vi "WILT Watering Times.vi"(5 "Watering Times Input":T3, 7 "Execution Type":enum16{"Write", "Read"}(ring), 8 "Error In":errorcluster, 11 "File Locations":T1[](array[typedef])) -> (0 "Error Out":errorcluster, 3 "Watering Times Output":T3)   [LabVIEW 2016]
uses:
  Type Definitions/WILT Injection Times.ctl
  Type Definitions/WILT Water Injection Control.ctl
  Utility/Save File/File Setup (Public)/Type Definition/Save File DOE File Path Control.ctl
  Utility/Save File/File Setup (Public)/Type Definition/Save File DOE Data Save Filepaths.ctl
  <vilib>/Utility/file.llb/Write To Spreadsheet File (string).vi
  <vilib>/Utility/file.llb/Read From Spreadsheet File (string).vi
  Utility/Save File/File Setup.lvlib
panel:
  out "all rows":string[][](array[string])
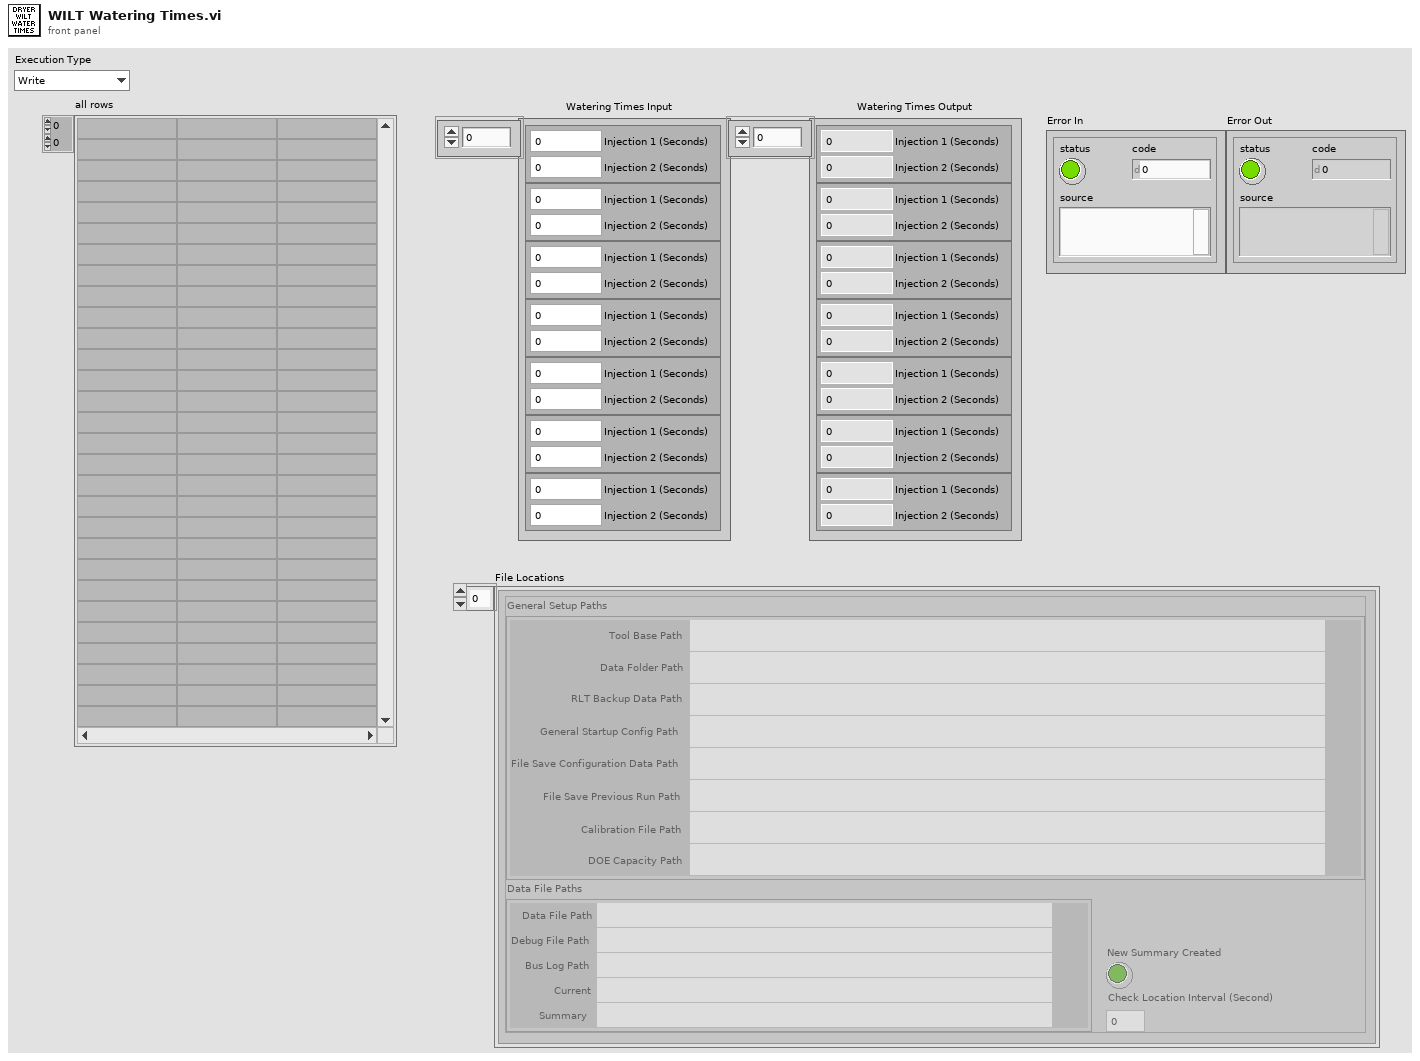
[diagram p1: front panel]
types:
  T1 = typedef "File Setup.lvlib/Save File DOE File Path Control.ctl" = cluster{"General Setup Paths":cluster{"Calibration File Path":path, "DOE Capacity Path":path, "Data Folder Path":path, "RLT Backup Data Path":path, "Tool Base Path":path, "General Startup Config Path":path, "File Save Previous Run Path":path, "File Save Configuration Data Path":path}, "Data File Paths":T2, "New Summary Created":bool, "Check Location Interval (Second)":i32}
  T2 = typedef "File Setup.lvlib/Save File DOE Data Save Filepaths.ctl" = cluster{"Data File Path":path, "Debug File Path":path, "Bus Log Path":path, "Current":path, "Summary":path}
  T3 = typedef "WILT Injection Times.ctl" = T4[]
  T4 = typedef "WILT Water Injection Control.ctl" = cluster{"Injection 1 (Seconds)":dbl, "Injection 2 (Seconds)":dbl}
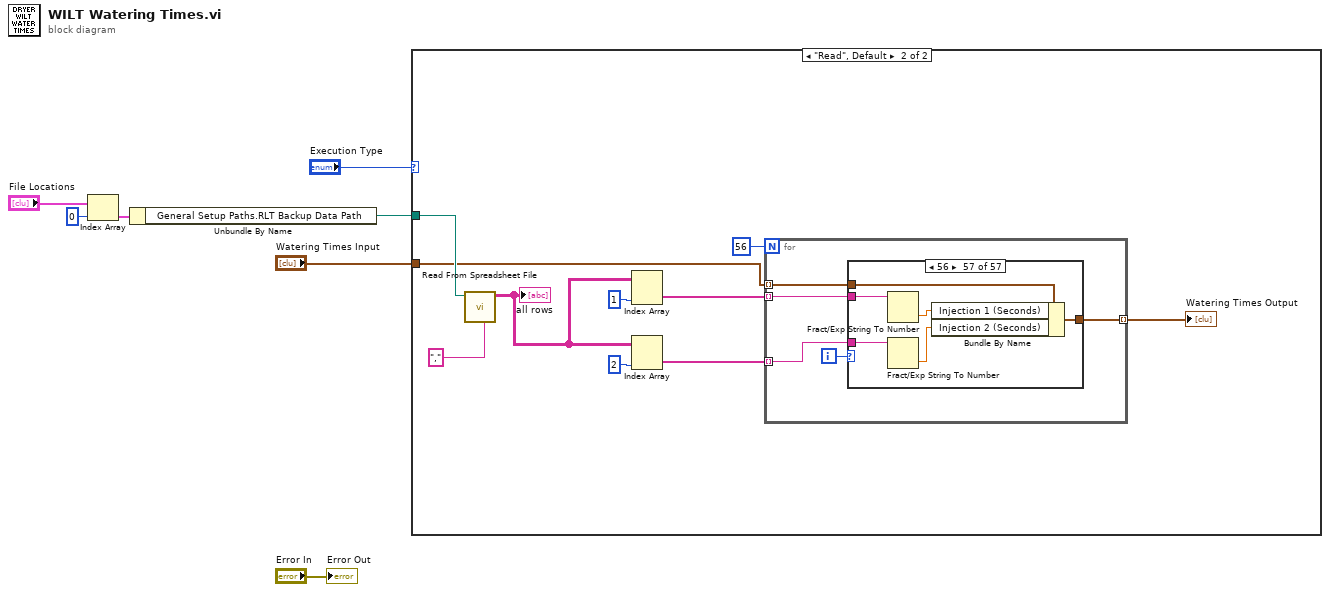
[diagram p0: block diagram]
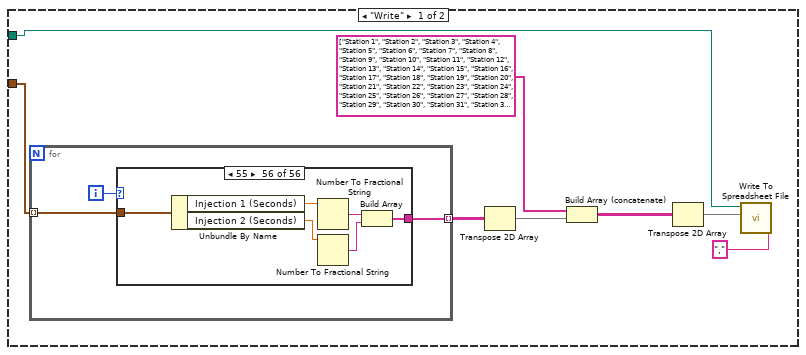
[diagram p2: hidden frame]
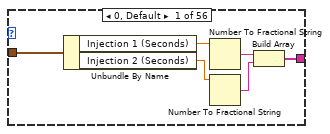
[diagram p3: hidden frame]
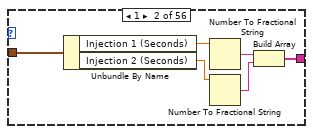
[diagram p4: hidden frame]
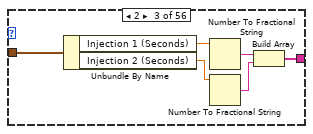
[diagram p5: hidden frame]
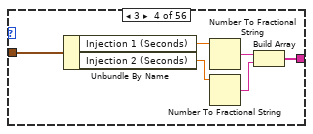
[diagram p6: hidden frame]
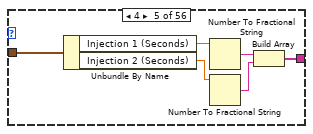
[diagram p7: hidden frame]
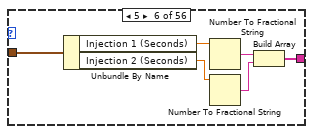
[diagram p8: hidden frame]
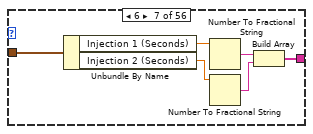
[diagram p9: hidden frame]
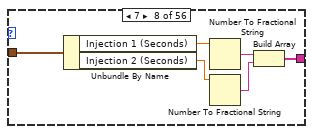
[diagram p10: hidden frame]
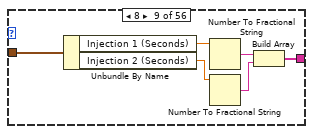
[diagram p11: hidden frame]
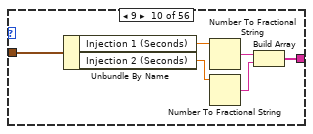
[diagram p12: hidden frame]
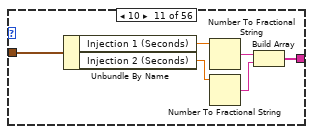
[diagram p13: hidden frame]
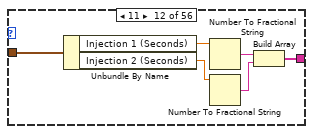
[diagram p14: hidden frame]
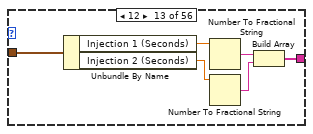
[diagram p15: hidden frame]
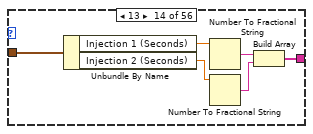
[diagram p16: hidden frame]
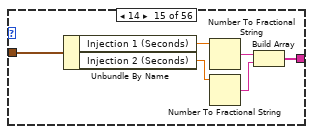
[diagram p17: hidden frame]
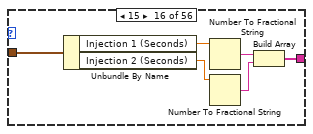
[diagram p18: hidden frame]
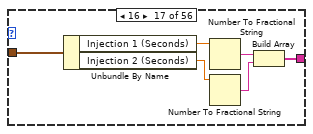
[diagram p19: hidden frame]
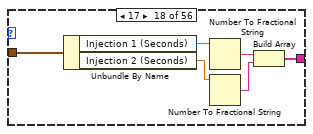
[diagram p20: hidden frame]
diagram:
  n1 = Index Array(array="File Locations", index=0) -> (element=w2:T1)
  n2 = Unbundle By Name(w2) -> ("General Setup Paths.RLT Backup Data Path"=w1:path)
  n3 = case shown="\"Read\", Default" "Execution Type" {
    tunnel: w1 -> [w10 w364]
    tunnel: "Watering Times Input" -> [w11 w356]
    frame "Write" {
      n4 = for {
        tunnel: w11 -> [w18] mode=indexing
        tunnel: [w17] -> w14 mode=indexing
        i -> [w16]
        n5 = case shown="55" w16 {
          tunnel: w18 -> [w24 w26 w32 w38 w43 w49 w55 w61 w67 w73 w79 w85 w91 w97 w103 w109 w115 w121 w127 w133 w139 w145 w151 w157 w163 w169 w175 w181 w187 w193 w199 w205 w211 w217 w223 w229 w235 w241 w247 w253 w259 w265 w271 w277 w283 w289 w295 w301 w307 w313 w319 w325 w331 w337 w343 w349]
          tunnel: [w19 w25 w31 w37 w44 w50 w56 w62 w68 w74 w80 w86 w92 w98 w104 w110 w116 w122 w128 w134 w140 w146 w152 w158 w164 w170 w176 w182 w188 w194 w200 w206 w212 w218 w224 w230 w236 w242 w248 w254 w260 w266 w272 w278 w284 w290 w296 w302 w308 w314 w320 w326 w332 w338 w344 w350] -> w17
          frame 0, Default {
            n6 = Unbundle By Name(w24) -> ("Injection 1 (Seconds)"=w23:dbl, "Injection 2 (Seconds)"=w22:dbl)
            n7 = Number To Fractional String(number=w23) -> (F-format string=w21:string)  [unwired: 3 in]
            n8 = Number To Fractional String(number=w22) -> (F-format string=w20:string)  [unwired: 3 in]
            n9 = Build Array(w21, w20) -> (w19:string[])
          }
          frame 1 {
            n10 = Unbundle By Name(w26) -> ("Injection 1 (Seconds)"=w30:dbl, "Injection 2 (Seconds)"=w29:dbl)
            n11 = Number To Fractional String(number=w30) -> (F-format string=w28:string)  [unwired: 3 in]
            n12 = Number To Fractional String(number=w29) -> (F-format string=w27:string)  [unwired: 3 in]
            n13 = Build Array(w28, w27) -> (w25:string[])
          }
          frame 2 {
            n14 = Unbundle By Name(w32) -> ("Injection 1 (Seconds)"=w36:dbl, "Injection 2 (Seconds)"=w35:dbl)
            n15 = Number To Fractional String(number=w36) -> (F-format string=w34:string)  [unwired: 3 in]
            n16 = Number To Fractional String(number=w35) -> (F-format string=w33:string)  [unwired: 3 in]
            n17 = Build Array(w34, w33) -> (w31:string[])
          }
          frame 3 {
            n18 = Unbundle By Name(w38) -> ("Injection 1 (Seconds)"=w42:dbl, "Injection 2 (Seconds)"=w41:dbl)
            n19 = Number To Fractional String(number=w42) -> (F-format string=w40:string)  [unwired: 3 in]
            n20 = Number To Fractional String(number=w41) -> (F-format string=w39:string)  [unwired: 3 in]
            n21 = Build Array(w40, w39) -> (w37:string[])
          }
          frame 4 {
            n22 = Unbundle By Name(w43) -> ("Injection 1 (Seconds)"=w48:dbl, "Injection 2 (Seconds)"=w47:dbl)
            n23 = Number To Fractional String(number=w48) -> (F-format string=w46:string)  [unwired: 3 in]
            n24 = Number To Fractional String(number=w47) -> (F-format string=w45:string)  [unwired: 3 in]
            n25 = Build Array(w46, w45) -> (w44:string[])
          }
          frame 5 {
            n26 = Unbundle By Name(w49) -> ("Injection 1 (Seconds)"=w54:dbl, "Injection 2 (Seconds)"=w53:dbl)
            n27 = Number To Fractional String(number=w54) -> (F-format string=w52:string)  [unwired: 3 in]
            n28 = Number To Fractional String(number=w53) -> (F-format string=w51:string)  [unwired: 3 in]
            n29 = Build Array(w52, w51) -> (w50:string[])
          }
          frame 6 {
            n30 = Unbundle By Name(w55) -> ("Injection 1 (Seconds)"=w60:dbl, "Injection 2 (Seconds)"=w59:dbl)
            n31 = Number To Fractional String(number=w60) -> (F-format string=w58:string)  [unwired: 3 in]
            n32 = Number To Fractional String(number=w59) -> (F-format string=w57:string)  [unwired: 3 in]
            n33 = Build Array(w58, w57) -> (w56:string[])
          }
          frame 7 {
            n34 = Unbundle By Name(w61) -> ("Injection 1 (Seconds)"=w66:dbl, "Injection 2 (Seconds)"=w65:dbl)
            n35 = Number To Fractional String(number=w66) -> (F-format string=w64:string)  [unwired: 3 in]
            n36 = Number To Fractional String(number=w65) -> (F-format string=w63:string)  [unwired: 3 in]
            n37 = Build Array(w64, w63) -> (w62:string[])
          }
          frame 8 {
            n38 = Unbundle By Name(w67) -> ("Injection 1 (Seconds)"=w72:dbl, "Injection 2 (Seconds)"=w71:dbl)
            n39 = Number To Fractional String(number=w72) -> (F-format string=w70:string)  [unwired: 3 in]
            n40 = Number To Fractional String(number=w71) -> (F-format string=w69:string)  [unwired: 3 in]
            n41 = Build Array(w70, w69) -> (w68:string[])
          }
          frame 9 {
            n42 = Unbundle By Name(w73) -> ("Injection 1 (Seconds)"=w78:dbl, "Injection 2 (Seconds)"=w77:dbl)
            n43 = Number To Fractional String(number=w78) -> (F-format string=w76:string)  [unwired: 3 in]
            n44 = Number To Fractional String(number=w77) -> (F-format string=w75:string)  [unwired: 3 in]
            n45 = Build Array(w76, w75) -> (w74:string[])
          }
          frame 10 {
            n46 = Unbundle By Name(w79) -> ("Injection 1 (Seconds)"=w84:dbl, "Injection 2 (Seconds)"=w83:dbl)
            n47 = Number To Fractional String(number=w84) -> (F-format string=w82:string)  [unwired: 3 in]
            n48 = Number To Fractional String(number=w83) -> (F-format string=w81:string)  [unwired: 3 in]
            n49 = Build Array(w82, w81) -> (w80:string[])
          }
          frame 11 {
            n50 = Unbundle By Name(w85) -> ("Injection 1 (Seconds)"=w90:dbl, "Injection 2 (Seconds)"=w89:dbl)
            n51 = Number To Fractional String(number=w90) -> (F-format string=w88:string)  [unwired: 3 in]
            n52 = Number To Fractional String(number=w89) -> (F-format string=w87:string)  [unwired: 3 in]
            n53 = Build Array(w88, w87) -> (w86:string[])
          }
          frame 12 {
            n54 = Unbundle By Name(w91) -> ("Injection 1 (Seconds)"=w96:dbl, "Injection 2 (Seconds)"=w95:dbl)
            n55 = Number To Fractional String(number=w96) -> (F-format string=w94:string)  [unwired: 3 in]
            n56 = Number To Fractional String(number=w95) -> (F-format string=w93:string)  [unwired: 3 in]
            n57 = Build Array(w94, w93) -> (w92:string[])
          }
          frame 13 {
            n58 = Unbundle By Name(w97) -> ("Injection 1 (Seconds)"=w102:dbl, "Injection 2 (Seconds)"=w101:dbl)
            n59 = Number To Fractional String(number=w102) -> (F-format string=w100:string)  [unwired: 3 in]
            n60 = Number To Fractional String(number=w101) -> (F-format string=w99:string)  [unwired: 3 in]
            n61 = Build Array(w100, w99) -> (w98:string[])
          }
          frame 14 {
            n62 = Unbundle By Name(w103) -> ("Injection 1 (Seconds)"=w108:dbl, "Injection 2 (Seconds)"=w107:dbl)
            n63 = Number To Fractional String(number=w108) -> (F-format string=w106:string)  [unwired: 3 in]
            n64 = Number To Fractional String(number=w107) -> (F-format string=w105:string)  [unwired: 3 in]
            n65 = Build Array(w106, w105) -> (w104:string[])
          }
          frame 15 {
            n66 = Unbundle By Name(w109) -> ("Injection 1 (Seconds)"=w114:dbl, "Injection 2 (Seconds)"=w113:dbl)
            n67 = Number To Fractional String(number=w114) -> (F-format string=w112:string)  [unwired: 3 in]
            n68 = Number To Fractional String(number=w113) -> (F-format string=w111:string)  [unwired: 3 in]
            n69 = Build Array(w112, w111) -> (w110:string[])
          }
          frame 16 {
            n70 = Unbundle By Name(w115) -> ("Injection 1 (Seconds)"=w120:dbl, "Injection 2 (Seconds)"=w119:dbl)
            n71 = Number To Fractional String(number=w120) -> (F-format string=w118:string)  [unwired: 3 in]
            n72 = Number To Fractional String(number=w119) -> (F-format string=w117:string)  [unwired: 3 in]
            n73 = Build Array(w118, w117) -> (w116:string[])
          }
          frame 17 {
            n74 = Unbundle By Name(w121) -> ("Injection 1 (Seconds)"=w126:dbl, "Injection 2 (Seconds)"=w125:dbl)
            n75 = Number To Fractional String(number=w126) -> (F-format string=w124:string)  [unwired: 3 in]
            n76 = Number To Fractional String(number=w125) -> (F-format string=w123:string)  [unwired: 3 in]
            n77 = Build Array(w124, w123) -> (w122:string[])
          }
          frame 18 {
            n78 = Unbundle By Name(w127) -> ("Injection 1 (Seconds)"=w132:dbl, "Injection 2 (Seconds)"=w131:dbl)
            n79 = Number To Fractional String(number=w132) -> (F-format string=w130:string)  [unwired: 3 in]
            n80 = Number To Fractional String(number=w131) -> (F-format string=w129:string)  [unwired: 3 in]
            n81 = Build Array(w130, w129) -> (w128:string[])
          }
          frame 19 {
            n82 = Unbundle By Name(w133) -> ("Injection 1 (Seconds)"=w138:dbl, "Injection 2 (Seconds)"=w137:dbl)
            n83 = Number To Fractional String(number=w138) -> (F-format string=w136:string)  [unwired: 3 in]
            n84 = Number To Fractional String(number=w137) -> (F-format string=w135:string)  [unwired: 3 in]
            n85 = Build Array(w136, w135) -> (w134:string[])
          }
          frame 20 {
            n86 = Unbundle By Name(w139) -> ("Injection 1 (Seconds)"=w144:dbl, "Injection 2 (Seconds)"=w143:dbl)
            n87 = Number To Fractional String(number=w144) -> (F-format string=w142:string)  [unwired: 3 in]
            n88 = Number To Fractional String(number=w143) -> (F-format string=w141:string)  [unwired: 3 in]
            n89 = Build Array(w142, w141) -> (w140:string[])
          }
          frame 21 {
            n90 = Unbundle By Name(w145) -> ("Injection 1 (Seconds)"=w150:dbl, "Injection 2 (Seconds)"=w149:dbl)
            n91 = Number To Fractional String(number=w150) -> (F-format string=w148:string)  [unwired: 3 in]
            n92 = Number To Fractional String(number=w149) -> (F-format string=w147:string)  [unwired: 3 in]
            n93 = Build Array(w148, w147) -> (w146:string[])
          }
          frame 22 {
            n94 = Unbundle By Name(w151) -> ("Injection 1 (Seconds)"=w156:dbl, "Injection 2 (Seconds)"=w155:dbl)
            n95 = Number To Fractional String(number=w156) -> (F-format string=w154:string)  [unwired: 3 in]
            n96 = Number To Fractional String(number=w155) -> (F-format string=w153:string)  [unwired: 3 in]
            n97 = Build Array(w154, w153) -> (w152:string[])
          }
          frame 23 {
            n98 = Unbundle By Name(w157) -> ("Injection 1 (Seconds)"=w162:dbl, "Injection 2 (Seconds)"=w161:dbl)
            n99 = Number To Fractional String(number=w162) -> (F-format string=w160:string)  [unwired: 3 in]
            n100 = Number To Fractional String(number=w161) -> (F-format string=w159:string)  [unwired: 3 in]
            n101 = Build Array(w160, w159) -> (w158:string[])
          }
          frame 24 {
            n102 = Unbundle By Name(w163) -> ("Injection 1 (Seconds)"=w168:dbl, "Injection 2 (Seconds)"=w167:dbl)
            n103 = Number To Fractional String(number=w168) -> (F-format string=w166:string)  [unwired: 3 in]
            n104 = Number To Fractional String(number=w167) -> (F-format string=w165:string)  [unwired: 3 in]
            n105 = Build Array(w166, w165) -> (w164:string[])
          }
          frame 25 {
            n106 = Unbundle By Name(w169) -> ("Injection 1 (Seconds)"=w174:dbl, "Injection 2 (Seconds)"=w173:dbl)
            n107 = Number To Fractional String(number=w174) -> (F-format string=w172:string)  [unwired: 3 in]
            n108 = Number To Fractional String(number=w173) -> (F-format string=w171:string)  [unwired: 3 in]
            n109 = Build Array(w172, w171) -> (w170:string[])
          }
          frame 26 {
            n110 = Unbundle By Name(w175) -> ("Injection 1 (Seconds)"=w180:dbl, "Injection 2 (Seconds)"=w179:dbl)
            n111 = Number To Fractional String(number=w180) -> (F-format string=w178:string)  [unwired: 3 in]
            n112 = Number To Fractional String(number=w179) -> (F-format string=w177:string)  [unwired: 3 in]
            n113 = Build Array(w178, w177) -> (w176:string[])
          }
          frame 27 {
            n114 = Unbundle By Name(w181) -> ("Injection 1 (Seconds)"=w186:dbl, "Injection 2 (Seconds)"=w185:dbl)
            n115 = Number To Fractional String(number=w186) -> (F-format string=w184:string)  [unwired: 3 in]
            n116 = Number To Fractional String(number=w185) -> (F-format string=w183:string)  [unwired: 3 in]
            n117 = Build Array(w184, w183) -> (w182:string[])
          }
          frame 28 {
            n118 = Unbundle By Name(w187) -> ("Injection 1 (Seconds)"=w192:dbl, "Injection 2 (Seconds)"=w191:dbl)
            n119 = Number To Fractional String(number=w192) -> (F-format string=w190:string)  [unwired: 3 in]
            n120 = Number To Fractional String(number=w191) -> (F-format string=w189:string)  [unwired: 3 in]
            n121 = Build Array(w190, w189) -> (w188:string[])
          }
          frame 29 {
            n122 = Unbundle By Name(w193) -> ("Injection 1 (Seconds)"=w198:dbl, "Injection 2 (Seconds)"=w197:dbl)
            n123 = Number To Fractional String(number=w198) -> (F-format string=w196:string)  [unwired: 3 in]
            n124 = Number To Fractional String(number=w197) -> (F-format string=w195:string)  [unwired: 3 in]
            n125 = Build Array(w196, w195) -> (w194:string[])
          }
          frame 30 {
            n126 = Unbundle By Name(w199) -> ("Injection 1 (Seconds)"=w204:dbl, "Injection 2 (Seconds)"=w203:dbl)
            n127 = Number To Fractional String(number=w204) -> (F-format string=w202:string)  [unwired: 3 in]
            n128 = Number To Fractional String(number=w203) -> (F-format string=w201:string)  [unwired: 3 in]
            n129 = Build Array(w202, w201) -> (w200:string[])
          }
          frame 31 {
            n130 = Unbundle By Name(w205) -> ("Injection 1 (Seconds)"=w210:dbl, "Injection 2 (Seconds)"=w209:dbl)
            n131 = Number To Fractional String(number=w210) -> (F-format string=w208:string)  [unwired: 3 in]
            n132 = Number To Fractional String(number=w209) -> (F-format string=w207:string)  [unwired: 3 in]
            n133 = Build Array(w208, w207) -> (w206:string[])
          }
          frame 32 {
            n134 = Unbundle By Name(w211) -> ("Injection 1 (Seconds)"=w216:dbl, "Injection 2 (Seconds)"=w215:dbl)
            n135 = Number To Fractional String(number=w216) -> (F-format string=w214:string)  [unwired: 3 in]
            n136 = Number To Fractional String(number=w215) -> (F-format string=w213:string)  [unwired: 3 in]
            n137 = Build Array(w214, w213) -> (w212:string[])
          }
          frame 33 {
            n138 = Unbundle By Name(w217) -> ("Injection 1 (Seconds)"=w222:dbl, "Injection 2 (Seconds)"=w221:dbl)
            n139 = Number To Fractional String(number=w222) -> (F-format string=w220:string)  [unwired: 3 in]
            n140 = Number To Fractional String(number=w221) -> (F-format string=w219:string)  [unwired: 3 in]
            n141 = Build Array(w220, w219) -> (w218:string[])
          }
          frame 34 {
            n142 = Unbundle By Name(w223) -> ("Injection 1 (Seconds)"=w228:dbl, "Injection 2 (Seconds)"=w227:dbl)
            n143 = Number To Fractional String(number=w228) -> (F-format string=w226:string)  [unwired: 3 in]
            n144 = Number To Fractional String(number=w227) -> (F-format string=w225:string)  [unwired: 3 in]
            n145 = Build Array(w226, w225) -> (w224:string[])
          }
          frame 35 {
            n146 = Unbundle By Name(w229) -> ("Injection 1 (Seconds)"=w234:dbl, "Injection 2 (Seconds)"=w233:dbl)
            n147 = Number To Fractional String(number=w234) -> (F-format string=w232:string)  [unwired: 3 in]
            n148 = Number To Fractional String(number=w233) -> (F-format string=w231:string)  [unwired: 3 in]
            n149 = Build Array(w232, w231) -> (w230:string[])
          }
          frame 36 {
            n150 = Unbundle By Name(w235) -> ("Injection 1 (Seconds)"=w240:dbl, "Injection 2 (Seconds)"=w239:dbl)
            n151 = Number To Fractional String(number=w240) -> (F-format string=w238:string)  [unwired: 3 in]
            n152 = Number To Fractional String(number=w239) -> (F-format string=w237:string)  [unwired: 3 in]
            n153 = Build Array(w238, w237) -> (w236:string[])
          }
          frame 37 {
            n154 = Unbundle By Name(w241) -> ("Injection 1 (Seconds)"=w246:dbl, "Injection 2 (Seconds)"=w245:dbl)
            n155 = Number To Fractional String(number=w246) -> (F-format string=w244:string)  [unwired: 3 in]
            n156 = Number To Fractional String(number=w245) -> (F-format string=w243:string)  [unwired: 3 in]
            n157 = Build Array(w244, w243) -> (w242:string[])
          }
          frame 38 {
            n158 = Unbundle By Name(w247) -> ("Injection 1 (Seconds)"=w252:dbl, "Injection 2 (Seconds)"=w251:dbl)
            n159 = Number To Fractional String(number=w252) -> (F-format string=w250:string)  [unwired: 3 in]
            n160 = Number To Fractional String(number=w251) -> (F-format string=w249:string)  [unwired: 3 in]
            n161 = Build Array(w250, w249) -> (w248:string[])
          }
          frame 39 {
            n162 = Unbundle By Name(w253) -> ("Injection 1 (Seconds)"=w258:dbl, "Injection 2 (Seconds)"=w257:dbl)
            n163 = Number To Fractional String(number=w258) -> (F-format string=w256:string)  [unwired: 3 in]
            n164 = Number To Fractional String(number=w257) -> (F-format string=w255:string)  [unwired: 3 in]
            n165 = Build Array(w256, w255) -> (w254:string[])
          }
          frame 40 {
            n166 = Unbundle By Name(w259) -> ("Injection 1 (Seconds)"=w264:dbl, "Injection 2 (Seconds)"=w263:dbl)
            n167 = Number To Fractional String(number=w264) -> (F-format string=w262:string)  [unwired: 3 in]
            n168 = Number To Fractional String(number=w263) -> (F-format string=w261:string)  [unwired: 3 in]
            n169 = Build Array(w262, w261) -> (w260:string[])
          }
          frame 41 {
            n170 = Unbundle By Name(w265) -> ("Injection 1 (Seconds)"=w270:dbl, "Injection 2 (Seconds)"=w269:dbl)
            n171 = Number To Fractional String(number=w270) -> (F-format string=w268:string)  [unwired: 3 in]
            n172 = Number To Fractional String(number=w269) -> (F-format string=w267:string)  [unwired: 3 in]
            n173 = Build Array(w268, w267) -> (w266:string[])
          }
          frame 42 {
            n174 = Unbundle By Name(w271) -> ("Injection 1 (Seconds)"=w276:dbl, "Injection 2 (Seconds)"=w275:dbl)
            n175 = Number To Fractional String(number=w276) -> (F-format string=w274:string)  [unwired: 3 in]
            n176 = Number To Fractional String(number=w275) -> (F-format string=w273:string)  [unwired: 3 in]
            n177 = Build Array(w274, w273) -> (w272:string[])
          }
          frame 43 {
            n178 = Unbundle By Name(w277) -> ("Injection 1 (Seconds)"=w282:dbl, "Injection 2 (Seconds)"=w281:dbl)
            n179 = Number To Fractional String(number=w282) -> (F-format string=w280:string)  [unwired: 3 in]
            n180 = Number To Fractional String(number=w281) -> (F-format string=w279:string)  [unwired: 3 in]
            n181 = Build Array(w280, w279) -> (w278:string[])
          }
          frame 44 {
            n182 = Unbundle By Name(w283) -> ("Injection 1 (Seconds)"=w288:dbl, "Injection 2 (Seconds)"=w287:dbl)
            n183 = Number To Fractional String(number=w288) -> (F-format string=w286:string)  [unwired: 3 in]
            n184 = Number To Fractional String(number=w287) -> (F-format string=w285:string)  [unwired: 3 in]
            n185 = Build Array(w286, w285) -> (w284:string[])
          }
          frame 45 {
            n186 = Unbundle By Name(w289) -> ("Injection 1 (Seconds)"=w294:dbl, "Injection 2 (Seconds)"=w293:dbl)
            n187 = Number To Fractional String(number=w294) -> (F-format string=w292:string)  [unwired: 3 in]
            n188 = Number To Fractional String(number=w293) -> (F-format string=w291:string)  [unwired: 3 in]
            n189 = Build Array(w292, w291) -> (w290:string[])
          }
          frame 46 {
            n190 = Unbundle By Name(w295) -> ("Injection 1 (Seconds)"=w300:dbl, "Injection 2 (Seconds)"=w299:dbl)
            n191 = Number To Fractional String(number=w300) -> (F-format string=w298:string)  [unwired: 3 in]
            n192 = Number To Fractional String(number=w299) -> (F-format string=w297:string)  [unwired: 3 in]
            n193 = Build Array(w298, w297) -> (w296:string[])
          }
          frame 47 {
            n194 = Unbundle By Name(w301) -> ("Injection 1 (Seconds)"=w306:dbl, "Injection 2 (Seconds)"=w305:dbl)
            n195 = Number To Fractional String(number=w306) -> (F-format string=w304:string)  [unwired: 3 in]
            n196 = Number To Fractional String(number=w305) -> (F-format string=w303:string)  [unwired: 3 in]
            n197 = Build Array(w304, w303) -> (w302:string[])
          }
          frame 48 {
            n198 = Unbundle By Name(w307) -> ("Injection 1 (Seconds)"=w312:dbl, "Injection 2 (Seconds)"=w311:dbl)
            n199 = Number To Fractional String(number=w312) -> (F-format string=w310:string)  [unwired: 3 in]
            n200 = Number To Fractional String(number=w311) -> (F-format string=w309:string)  [unwired: 3 in]
            n201 = Build Array(w310, w309) -> (w308:string[])
          }
          frame 49 {
            n202 = Unbundle By Name(w313) -> ("Injection 1 (Seconds)"=w318:dbl, "Injection 2 (Seconds)"=w317:dbl)
            n203 = Number To Fractional String(number=w318) -> (F-format string=w316:string)  [unwired: 3 in]
            n204 = Number To Fractional String(number=w317) -> (F-format string=w315:string)  [unwired: 3 in]
            n205 = Build Array(w316, w315) -> (w314:string[])
          }
          frame 50 {
            n206 = Unbundle By Name(w319) -> ("Injection 1 (Seconds)"=w324:dbl, "Injection 2 (Seconds)"=w323:dbl)
            n207 = Number To Fractional String(number=w324) -> (F-format string=w322:string)  [unwired: 3 in]
            n208 = Number To Fractional String(number=w323) -> (F-format string=w321:string)  [unwired: 3 in]
            n209 = Build Array(w322, w321) -> (w320:string[])
          }
          frame 51 {
            n210 = Unbundle By Name(w325) -> ("Injection 1 (Seconds)"=w330:dbl, "Injection 2 (Seconds)"=w329:dbl)
            n211 = Number To Fractional String(number=w330) -> (F-format string=w328:string)  [unwired: 3 in]
            n212 = Number To Fractional String(number=w329) -> (F-format string=w327:string)  [unwired: 3 in]
            n213 = Build Array(w328, w327) -> (w326:string[])
          }
          frame 52 {
            n214 = Unbundle By Name(w331) -> ("Injection 1 (Seconds)"=w336:dbl, "Injection 2 (Seconds)"=w335:dbl)
            n215 = Number To Fractional String(number=w336) -> (F-format string=w334:string)  [unwired: 3 in]
            n216 = Number To Fractional String(number=w335) -> (F-format string=w333:string)  [unwired: 3 in]
            n217 = Build Array(w334, w333) -> (w332:string[])
          }
          frame 53 {
            n218 = Unbundle By Name(w337) -> ("Injection 1 (Seconds)"=w342:dbl, "Injection 2 (Seconds)"=w341:dbl)
            n219 = Number To Fractional String(number=w342) -> (F-format string=w340:string)  [unwired: 3 in]
            n220 = Number To Fractional String(number=w341) -> (F-format string=w339:string)  [unwired: 3 in]
            n221 = Build Array(w340, w339) -> (w338:string[])
          }
          frame 54 {
            n222 = Unbundle By Name(w343) -> ("Injection 1 (Seconds)"=w348:dbl, "Injection 2 (Seconds)"=w347:dbl)
            n223 = Number To Fractional String(number=w348) -> (F-format string=w346:string)  [unwired: 3 in]
            n224 = Number To Fractional String(number=w347) -> (F-format string=w345:string)  [unwired: 3 in]
            n225 = Build Array(w346, w345) -> (w344:string[])
          }
          frame 55 {
            n226 = Unbundle By Name(w349) -> ("Injection 1 (Seconds)"=w354:dbl, "Injection 2 (Seconds)"=w353:dbl)
            n227 = Number To Fractional String(number=w354) -> (F-format string=w352:string)  [unwired: 3 in]
            n228 = Number To Fractional String(number=w353) -> (F-format string=w351:string)  [unwired: 3 in]
            n229 = Build Array(w352, w351) -> (w350:string[])
          }
        }
      }
      n230 = Transpose 2D Array(2D array=w14) -> (transposed array=w15:string[][])
      n231 = Build Array (concatenate)(string[] ["Station 1", "Station 2", "Station 3", "Station 4", "Station 5", "Station 6", "Station 7", "Station 8", "Station 9", "Station 10", "Station 11", "Station 12", "Station 13", "Station 14", "Station 15", "Station 16", "Station 17", "Station 18", "Station 19", "Station 20", "Station 21", "Station 22", "Station 23", "Station 24", "Station 25", "Station 26", "Station 27", "Station 28", "Station 29", "Station 30", "Station 31", "Station 32", "Station 33", "Station 34", "Station 35", "Station 36", "Station 37", "Station 38", "Station 39", "Station 40", "Station 41", "Station 42", "Station 43", "Station 44", "Station 45", "Station 46", "Station 47", "Station 48", "Station 49", "Station 50", "Station 51", "Station 52", "Station 53", "Station 54", "Station 55", "Station 56"] ("subarray"), w15) -> (w13:string[][])
      n232 = Transpose 2D Array(2D array=w13) -> (transposed array=w9:string[][])
      n233 = call-poly <vilib>:"Write To Spreadsheet File.vi"("delimiter (\\t)"="," ("delimiter (\\t)"), "2D data"=w9, "file path (dialog if empty)"=w10) -> ()  [unwired: 5 in, 1 out]
    }
    frame "Read", Default {
      n234 = call-poly <vilib>:"Read From Spreadsheet File.vi"("delimiter (\\t)"="," ("delimiter (\\t)"), "file path (dialog if empty)"=w364) -> ("all rows"=w359:string[][])  [unwired: 5 in, 4 out]
      "all rows" <- w359
      n235 = Index Array(array=w359, index (col)=1 ("disabled index (col)")) -> (element=w361:string[])  [unwired: 1 in]
      n236 = Index Array(array=w359, index (col)=2 ("disabled index (col)")) -> (element=w358:string[])  [unwired: 1 in]
      n237 = for {
        N: 56 -> [_]
        tunnel: w361 -> [w366] mode=indexing
        tunnel: w356 -> [w368] mode=indexing
        tunnel: [w367] -> w355 mode=indexing
        tunnel: w358 -> [w365] mode=indexing
        i -> [w369]
        n238 = case shown="56" w369 {
          tunnel: w368 -> [w375 w379 w383 w391 w395 w403 w409 w415 w421 w427 w431 w437 w445 w451 w457 w463 w467 w473 w479 w485 w491 w497 w503 w509 w515 w521 w527 w533 w539 w545 w551 w559 w563 w569 w575 w581 w587 w593 w599 w605 w611 w617 w623 w629 w635 w641 w647 w653 w659 w665 w671 w677 w683 w689 w695 w701 w707]
          tunnel: [w374 w378 w382 w390 w394 w402 w408 w414 w420 w426 w430 w436 w444 w450 w456 w462 w466 w472 w478 w484 w490 w496 w502 w508 w514 w520 w526 w532 w538 w544 w550 w556 w562 w568 w574 w580 w586 w592 w598 w604 w610 w616 w622 w628 w634 w640 w646 w652 w658 w664 w670 w676 w682 w688 w694 w700 w706] -> w367
          tunnel: w366 -> [w373 w377 w385 w389 w396 w401 w407 w413 w419 w425 w433 w438 w443 w449 w455 w461 w469 w474 w480 w486 w492 w498 w505 w510 w516 w522 w528 w534 w541 w547 w553 w558 w565 w570 w577 w582 w588 w594 w600 w606 w612 w618 w624 w630 w637 w643 w649 w655 w661 w667 w673 w679 w685 w690 w696 w702 w709]
          tunnel: w365 -> [w371 w376 w384 w388 w397 w400 w406 w412 w418 w424 w432 w439 w442 w448 w454 w460 w468 w475 w481 w487 w493 w499 w504 w511 w517 w523 w529 w535 w540 w546 w552 w557 w564 w571 w576 w583 w589 w595 w601 w607 w613 w619 w625 w631 w636 w642 w648 w654 w660 w666 w672 w678 w684 w691 w697 w703 w708]
          frame 0, Default {
            n239 = Fract/Exp String To Number(string=w373) -> (number=w372:dbl)  [unwired: 3 in, 1 out]
            n240 = Fract/Exp String To Number(string=w371) -> (number=w370:dbl)  [unwired: 3 in, 1 out]
            n241 = Bundle By Name(cluster=w375, "Injection 1 (Seconds)"=w372, "Injection 2 (Seconds)"=w370) -> (w374:T4)
          }
          frame 1 {
            n242 = Fract/Exp String To Number(string=w377) -> (number=w381:dbl)  [unwired: 3 in, 1 out]
            n243 = Fract/Exp String To Number(string=w376) -> (number=w380:dbl)  [unwired: 3 in, 1 out]
            n244 = Bundle By Name(cluster=w379, "Injection 1 (Seconds)"=w381, "Injection 2 (Seconds)"=w380) -> (w378:T4)
          }
          frame 2 {
            n245 = Fract/Exp String To Number(string=w385) -> (number=w387:dbl)  [unwired: 3 in, 1 out]
            n246 = Fract/Exp String To Number(string=w384) -> (number=w386:dbl)  [unwired: 3 in, 1 out]
            n247 = Bundle By Name(cluster=w383, "Injection 1 (Seconds)"=w387, "Injection 2 (Seconds)"=w386) -> (w382:T4)
          }
          frame 3 {
            n248 = Fract/Exp String To Number(string=w389) -> (number=w393:dbl)  [unwired: 3 in, 1 out]
            n249 = Fract/Exp String To Number(string=w388) -> (number=w392:dbl)  [unwired: 3 in, 1 out]
            n250 = Bundle By Name(cluster=w391, "Injection 1 (Seconds)"=w393, "Injection 2 (Seconds)"=w392) -> (w390:T4)
          }
          frame 4 {
            n251 = Fract/Exp String To Number(string=w396) -> (number=w399:dbl)  [unwired: 3 in, 1 out]
            n252 = Fract/Exp String To Number(string=w397) -> (number=w398:dbl)  [unwired: 3 in, 1 out]
            n253 = Bundle By Name(cluster=w395, "Injection 1 (Seconds)"=w399, "Injection 2 (Seconds)"=w398) -> (w394:T4)
          }
          frame 5 {
            n254 = Fract/Exp String To Number(string=w401) -> (number=w405:dbl)  [unwired: 3 in, 1 out]
            n255 = Fract/Exp String To Number(string=w400) -> (number=w404:dbl)  [unwired: 3 in, 1 out]
            n256 = Bundle By Name(cluster=w403, "Injection 1 (Seconds)"=w405, "Injection 2 (Seconds)"=w404) -> (w402:T4)
          }
          frame 6 {
            n257 = Fract/Exp String To Number(string=w407) -> (number=w411:dbl)  [unwired: 3 in, 1 out]
            n258 = Fract/Exp String To Number(string=w406) -> (number=w410:dbl)  [unwired: 3 in, 1 out]
            n259 = Bundle By Name(cluster=w409, "Injection 1 (Seconds)"=w411, "Injection 2 (Seconds)"=w410) -> (w408:T4)
          }
          frame 7 {
            n260 = Fract/Exp String To Number(string=w413) -> (number=w417:dbl)  [unwired: 3 in, 1 out]
            n261 = Fract/Exp String To Number(string=w412) -> (number=w416:dbl)  [unwired: 3 in, 1 out]
            n262 = Bundle By Name(cluster=w415, "Injection 1 (Seconds)"=w417, "Injection 2 (Seconds)"=w416) -> (w414:T4)
          }
          frame 8 {
            n263 = Fract/Exp String To Number(string=w419) -> (number=w423:dbl)  [unwired: 3 in, 1 out]
            n264 = Fract/Exp String To Number(string=w418) -> (number=w422:dbl)  [unwired: 3 in, 1 out]
            n265 = Bundle By Name(cluster=w421, "Injection 1 (Seconds)"=w423, "Injection 2 (Seconds)"=w422) -> (w420:T4)
          }
          frame 9 {
            n266 = Fract/Exp String To Number(string=w425) -> (number=w429:dbl)  [unwired: 3 in, 1 out]
            n267 = Fract/Exp String To Number(string=w424) -> (number=w428:dbl)  [unwired: 3 in, 1 out]
            n268 = Bundle By Name(cluster=w427, "Injection 1 (Seconds)"=w429, "Injection 2 (Seconds)"=w428) -> (w426:T4)
          }
          frame 10 {
            n269 = Fract/Exp String To Number(string=w433) -> (number=w435:dbl)  [unwired: 3 in, 1 out]
            n270 = Fract/Exp String To Number(string=w432) -> (number=w434:dbl)  [unwired: 3 in, 1 out]
            n271 = Bundle By Name(cluster=w431, "Injection 1 (Seconds)"=w435, "Injection 2 (Seconds)"=w434) -> (w430:T4)
          }
          frame 11 {
            n272 = Fract/Exp String To Number(string=w438) -> (number=w441:dbl)  [unwired: 3 in, 1 out]
            n273 = Fract/Exp String To Number(string=w439) -> (number=w440:dbl)  [unwired: 3 in, 1 out]
            n274 = Bundle By Name(cluster=w437, "Injection 1 (Seconds)"=w441, "Injection 2 (Seconds)"=w440) -> (w436:T4)
          }
          frame 12 {
            n275 = Fract/Exp String To Number(string=w443) -> (number=w447:dbl)  [unwired: 3 in, 1 out]
            n276 = Fract/Exp String To Number(string=w442) -> (number=w446:dbl)  [unwired: 3 in, 1 out]
            n277 = Bundle By Name(cluster=w445, "Injection 1 (Seconds)"=w447, "Injection 2 (Seconds)"=w446) -> (w444:T4)
          }
          frame 13 {
            n278 = Fract/Exp String To Number(string=w449) -> (number=w453:dbl)  [unwired: 3 in, 1 out]
            n279 = Fract/Exp String To Number(string=w448) -> (number=w452:dbl)  [unwired: 3 in, 1 out]
            n280 = Bundle By Name(cluster=w451, "Injection 1 (Seconds)"=w453, "Injection 2 (Seconds)"=w452) -> (w450:T4)
          }
          frame 14 {
            n281 = Fract/Exp String To Number(string=w455) -> (number=w459:dbl)  [unwired: 3 in, 1 out]
            n282 = Fract/Exp String To Number(string=w454) -> (number=w458:dbl)  [unwired: 3 in, 1 out]
            n283 = Bundle By Name(cluster=w457, "Injection 1 (Seconds)"=w459, "Injection 2 (Seconds)"=w458) -> (w456:T4)
          }
          frame 15 {
            n284 = Fract/Exp String To Number(string=w461) -> (number=w465:dbl)  [unwired: 3 in, 1 out]
            n285 = Fract/Exp String To Number(string=w460) -> (number=w464:dbl)  [unwired: 3 in, 1 out]
            n286 = Bundle By Name(cluster=w463, "Injection 1 (Seconds)"=w465, "Injection 2 (Seconds)"=w464) -> (w462:T4)
          }
          frame 16 {
            n287 = Fract/Exp String To Number(string=w469) -> (number=w471:dbl)  [unwired: 3 in, 1 out]
            n288 = Fract/Exp String To Number(string=w468) -> (number=w470:dbl)  [unwired: 3 in, 1 out]
            n289 = Bundle By Name(cluster=w467, "Injection 1 (Seconds)"=w471, "Injection 2 (Seconds)"=w470) -> (w466:T4)
          }
          frame 17 {
            n290 = Fract/Exp String To Number(string=w474) -> (number=w477:dbl)  [unwired: 3 in, 1 out]
            n291 = Fract/Exp String To Number(string=w475) -> (number=w476:dbl)  [unwired: 3 in, 1 out]
            n292 = Bundle By Name(cluster=w473, "Injection 1 (Seconds)"=w477, "Injection 2 (Seconds)"=w476) -> (w472:T4)
          }
          frame 18 {
            n293 = Fract/Exp String To Number(string=w480) -> (number=w483:dbl)  [unwired: 3 in, 1 out]
            n294 = Fract/Exp String To Number(string=w481) -> (number=w482:dbl)  [unwired: 3 in, 1 out]
            n295 = Bundle By Name(cluster=w479, "Injection 1 (Seconds)"=w483, "Injection 2 (Seconds)"=w482) -> (w478:T4)
          }
          frame 19 {
            n296 = Fract/Exp String To Number(string=w486) -> (number=w489:dbl)  [unwired: 3 in, 1 out]
            n297 = Fract/Exp String To Number(string=w487) -> (number=w488:dbl)  [unwired: 3 in, 1 out]
            n298 = Bundle By Name(cluster=w485, "Injection 1 (Seconds)"=w489, "Injection 2 (Seconds)"=w488) -> (w484:T4)
          }
          frame 20 {
            n299 = Fract/Exp String To Number(string=w492) -> (number=w495:dbl)  [unwired: 3 in, 1 out]
            n300 = Fract/Exp String To Number(string=w493) -> (number=w494:dbl)  [unwired: 3 in, 1 out]
            n301 = Bundle By Name(cluster=w491, "Injection 1 (Seconds)"=w495, "Injection 2 (Seconds)"=w494) -> (w490:T4)
          }
          frame 21 {
            n302 = Fract/Exp String To Number(string=w498) -> (number=w501:dbl)  [unwired: 3 in, 1 out]
            n303 = Fract/Exp String To Number(string=w499) -> (number=w500:dbl)  [unwired: 3 in, 1 out]
            n304 = Bundle By Name(cluster=w497, "Injection 1 (Seconds)"=w501, "Injection 2 (Seconds)"=w500) -> (w496:T4)
          }
          frame 22 {
            n305 = Fract/Exp String To Number(string=w505) -> (number=w507:dbl)  [unwired: 3 in, 1 out]
            n306 = Fract/Exp String To Number(string=w504) -> (number=w506:dbl)  [unwired: 3 in, 1 out]
            n307 = Bundle By Name(cluster=w503, "Injection 1 (Seconds)"=w507, "Injection 2 (Seconds)"=w506) -> (w502:T4)
          }
          frame 23 {
            n308 = Fract/Exp String To Number(string=w510) -> (number=w513:dbl)  [unwired: 3 in, 1 out]
            n309 = Fract/Exp String To Number(string=w511) -> (number=w512:dbl)  [unwired: 3 in, 1 out]
            n310 = Bundle By Name(cluster=w509, "Injection 1 (Seconds)"=w513, "Injection 2 (Seconds)"=w512) -> (w508:T4)
          }
          frame 24 {
            n311 = Fract/Exp String To Number(string=w516) -> (number=w519:dbl)  [unwired: 3 in, 1 out]
            n312 = Fract/Exp String To Number(string=w517) -> (number=w518:dbl)  [unwired: 3 in, 1 out]
            n313 = Bundle By Name(cluster=w515, "Injection 1 (Seconds)"=w519, "Injection 2 (Seconds)"=w518) -> (w514:T4)
          }
          frame 25 {
            n314 = Fract/Exp String To Number(string=w522) -> (number=w525:dbl)  [unwired: 3 in, 1 out]
            n315 = Fract/Exp String To Number(string=w523) -> (number=w524:dbl)  [unwired: 3 in, 1 out]
            n316 = Bundle By Name(cluster=w521, "Injection 1 (Seconds)"=w525, "Injection 2 (Seconds)"=w524) -> (w520:T4)
          }
          frame 26 {
            n317 = Fract/Exp String To Number(string=w528) -> (number=w531:dbl)  [unwired: 3 in, 1 out]
            n318 = Fract/Exp String To Number(string=w529) -> (number=w530:dbl)  [unwired: 3 in, 1 out]
            n319 = Bundle By Name(cluster=w527, "Injection 1 (Seconds)"=w531, "Injection 2 (Seconds)"=w530) -> (w526:T4)
          }
          frame 27 {
            n320 = Fract/Exp String To Number(string=w534) -> (number=w537:dbl)  [unwired: 3 in, 1 out]
            n321 = Fract/Exp String To Number(string=w535) -> (number=w536:dbl)  [unwired: 3 in, 1 out]
            n322 = Bundle By Name(cluster=w533, "Injection 1 (Seconds)"=w537, "Injection 2 (Seconds)"=w536) -> (w532:T4)
          }
          frame 28 {
            n323 = Fract/Exp String To Number(string=w541) -> (number=w543:dbl)  [unwired: 3 in, 1 out]
            n324 = Fract/Exp String To Number(string=w540) -> (number=w542:dbl)  [unwired: 3 in, 1 out]
            n325 = Bundle By Name(cluster=w539, "Injection 1 (Seconds)"=w543, "Injection 2 (Seconds)"=w542) -> (w538:T4)
          }
          frame 29 {
            n326 = Fract/Exp String To Number(string=w547) -> (number=w549:dbl)  [unwired: 3 in, 1 out]
            n327 = Fract/Exp String To Number(string=w546) -> (number=w548:dbl)  [unwired: 3 in, 1 out]
            n328 = Bundle By Name(cluster=w545, "Injection 1 (Seconds)"=w549, "Injection 2 (Seconds)"=w548) -> (w544:T4)
          }
          frame 30 {
            n329 = Fract/Exp String To Number(string=w553) -> (number=w555:dbl)  [unwired: 3 in, 1 out]
            n330 = Fract/Exp String To Number(string=w552) -> (number=w554:dbl)  [unwired: 3 in, 1 out]
            n331 = Bundle By Name(cluster=w551, "Injection 1 (Seconds)"=w555, "Injection 2 (Seconds)"=w554) -> (w550:T4)
          }
          frame 31 {
            n332 = Fract/Exp String To Number(string=w558) -> (number=w561:dbl)  [unwired: 3 in, 1 out]
            n333 = Fract/Exp String To Number(string=w557) -> (number=w560:dbl)  [unwired: 3 in, 1 out]
            n334 = Bundle By Name(cluster=w559, "Injection 1 (Seconds)"=w561, "Injection 2 (Seconds)"=w560) -> (w556:T4)
          }
          frame 32 {
            n335 = Fract/Exp String To Number(string=w565) -> (number=w567:dbl)  [unwired: 3 in, 1 out]
            n336 = Fract/Exp String To Number(string=w564) -> (number=w566:dbl)  [unwired: 3 in, 1 out]
            n337 = Bundle By Name(cluster=w563, "Injection 1 (Seconds)"=w567, "Injection 2 (Seconds)"=w566) -> (w562:T4)
          }
          frame 33 {
            n338 = Fract/Exp String To Number(string=w570) -> (number=w573:dbl)  [unwired: 3 in, 1 out]
            n339 = Fract/Exp String To Number(string=w571) -> (number=w572:dbl)  [unwired: 3 in, 1 out]
            n340 = Bundle By Name(cluster=w569, "Injection 1 (Seconds)"=w573, "Injection 2 (Seconds)"=w572) -> (w568:T4)
          }
          frame 34 {
            n341 = Fract/Exp String To Number(string=w577) -> (number=w579:dbl)  [unwired: 3 in, 1 out]
            n342 = Fract/Exp String To Number(string=w576) -> (number=w578:dbl)  [unwired: 3 in, 1 out]
            n343 = Bundle By Name(cluster=w575, "Injection 1 (Seconds)"=w579, "Injection 2 (Seconds)"=w578) -> (w574:T4)
          }
          frame 35 {
            n344 = Fract/Exp String To Number(string=w582) -> (number=w585:dbl)  [unwired: 3 in, 1 out]
            n345 = Fract/Exp String To Number(string=w583) -> (number=w584:dbl)  [unwired: 3 in, 1 out]
            n346 = Bundle By Name(cluster=w581, "Injection 1 (Seconds)"=w585, "Injection 2 (Seconds)"=w584) -> (w580:T4)
          }
          frame 36 {
            n347 = Fract/Exp String To Number(string=w588) -> (number=w591:dbl)  [unwired: 3 in, 1 out]
            n348 = Fract/Exp String To Number(string=w589) -> (number=w590:dbl)  [unwired: 3 in, 1 out]
            n349 = Bundle By Name(cluster=w587, "Injection 1 (Seconds)"=w591, "Injection 2 (Seconds)"=w590) -> (w586:T4)
          }
          frame 37 {
            n350 = Fract/Exp String To Number(string=w594) -> (number=w597:dbl)  [unwired: 3 in, 1 out]
            n351 = Fract/Exp String To Number(string=w595) -> (number=w596:dbl)  [unwired: 3 in, 1 out]
            n352 = Bundle By Name(cluster=w593, "Injection 1 (Seconds)"=w597, "Injection 2 (Seconds)"=w596) -> (w592:T4)
          }
          frame 38 {
            n353 = Fract/Exp String To Number(string=w600) -> (number=w603:dbl)  [unwired: 3 in, 1 out]
            n354 = Fract/Exp String To Number(string=w601) -> (number=w602:dbl)  [unwired: 3 in, 1 out]
            n355 = Bundle By Name(cluster=w599, "Injection 1 (Seconds)"=w603, "Injection 2 (Seconds)"=w602) -> (w598:T4)
          }
          frame 39 {
            n356 = Fract/Exp String To Number(string=w606) -> (number=w609:dbl)  [unwired: 3 in, 1 out]
            n357 = Fract/Exp String To Number(string=w607) -> (number=w608:dbl)  [unwired: 3 in, 1 out]
            n358 = Bundle By Name(cluster=w605, "Injection 1 (Seconds)"=w609, "Injection 2 (Seconds)"=w608) -> (w604:T4)
          }
          frame 40 {
            n359 = Fract/Exp String To Number(string=w612) -> (number=w615:dbl)  [unwired: 3 in, 1 out]
            n360 = Fract/Exp String To Number(string=w613) -> (number=w614:dbl)  [unwired: 3 in, 1 out]
            n361 = Bundle By Name(cluster=w611, "Injection 1 (Seconds)"=w615, "Injection 2 (Seconds)"=w614) -> (w610:T4)
          }
          frame 41 {
            n362 = Fract/Exp String To Number(string=w618) -> (number=w621:dbl)  [unwired: 3 in, 1 out]
            n363 = Fract/Exp String To Number(string=w619) -> (number=w620:dbl)  [unwired: 3 in, 1 out]
            n364 = Bundle By Name(cluster=w617, "Injection 1 (Seconds)"=w621, "Injection 2 (Seconds)"=w620) -> (w616:T4)
          }
          frame 42 {
            n365 = Fract/Exp String To Number(string=w624) -> (number=w627:dbl)  [unwired: 3 in, 1 out]
            n366 = Fract/Exp String To Number(string=w625) -> (number=w626:dbl)  [unwired: 3 in, 1 out]
            n367 = Bundle By Name(cluster=w623, "Injection 1 (Seconds)"=w627, "Injection 2 (Seconds)"=w626) -> (w622:T4)
          }
          frame 43 {
            n368 = Fract/Exp String To Number(string=w630) -> (number=w633:dbl)  [unwired: 3 in, 1 out]
            n369 = Fract/Exp String To Number(string=w631) -> (number=w632:dbl)  [unwired: 3 in, 1 out]
            n370 = Bundle By Name(cluster=w629, "Injection 1 (Seconds)"=w633, "Injection 2 (Seconds)"=w632) -> (w628:T4)
          }
          frame 44 {
            n371 = Fract/Exp String To Number(string=w637) -> (number=w639:dbl)  [unwired: 3 in, 1 out]
            n372 = Fract/Exp String To Number(string=w636) -> (number=w638:dbl)  [unwired: 3 in, 1 out]
            n373 = Bundle By Name(cluster=w635, "Injection 1 (Seconds)"=w639, "Injection 2 (Seconds)"=w638) -> (w634:T4)
          }
          frame 45 {
            n374 = Fract/Exp String To Number(string=w643) -> (number=w645:dbl)  [unwired: 3 in, 1 out]
            n375 = Fract/Exp String To Number(string=w642) -> (number=w644:dbl)  [unwired: 3 in, 1 out]
            n376 = Bundle By Name(cluster=w641, "Injection 1 (Seconds)"=w645, "Injection 2 (Seconds)"=w644) -> (w640:T4)
          }
          frame 46 {
            n377 = Fract/Exp String To Number(string=w649) -> (number=w651:dbl)  [unwired: 3 in, 1 out]
            n378 = Fract/Exp String To Number(string=w648) -> (number=w650:dbl)  [unwired: 3 in, 1 out]
            n379 = Bundle By Name(cluster=w647, "Injection 1 (Seconds)"=w651, "Injection 2 (Seconds)"=w650) -> (w646:T4)
          }
          frame 47 {
            n380 = Fract/Exp String To Number(string=w655) -> (number=w657:dbl)  [unwired: 3 in, 1 out]
            n381 = Fract/Exp String To Number(string=w654) -> (number=w656:dbl)  [unwired: 3 in, 1 out]
            n382 = Bundle By Name(cluster=w653, "Injection 1 (Seconds)"=w657, "Injection 2 (Seconds)"=w656) -> (w652:T4)
          }
          frame 48 {
            n383 = Fract/Exp String To Number(string=w661) -> (number=w663:dbl)  [unwired: 3 in, 1 out]
            n384 = Fract/Exp String To Number(string=w660) -> (number=w662:dbl)  [unwired: 3 in, 1 out]
            n385 = Bundle By Name(cluster=w659, "Injection 1 (Seconds)"=w663, "Injection 2 (Seconds)"=w662) -> (w658:T4)
          }
          frame 49 {
            n386 = Fract/Exp String To Number(string=w667) -> (number=w669:dbl)  [unwired: 3 in, 1 out]
            n387 = Fract/Exp String To Number(string=w666) -> (number=w668:dbl)  [unwired: 3 in, 1 out]
            n388 = Bundle By Name(cluster=w665, "Injection 1 (Seconds)"=w669, "Injection 2 (Seconds)"=w668) -> (w664:T4)
          }
          frame 50 {
            n389 = Fract/Exp String To Number(string=w673) -> (number=w675:dbl)  [unwired: 3 in, 1 out]
            n390 = Fract/Exp String To Number(string=w672) -> (number=w674:dbl)  [unwired: 3 in, 1 out]
            n391 = Bundle By Name(cluster=w671, "Injection 1 (Seconds)"=w675, "Injection 2 (Seconds)"=w674) -> (w670:T4)
          }
          frame 51 {
            n392 = Fract/Exp String To Number(string=w679) -> (number=w681:dbl)  [unwired: 3 in, 1 out]
            n393 = Fract/Exp String To Number(string=w678) -> (number=w680:dbl)  [unwired: 3 in, 1 out]
            n394 = Bundle By Name(cluster=w677, "Injection 1 (Seconds)"=w681, "Injection 2 (Seconds)"=w680) -> (w676:T4)
          }
          frame 52 {
            n395 = Fract/Exp String To Number(string=w685) -> (number=w687:dbl)  [unwired: 3 in, 1 out]
            n396 = Fract/Exp String To Number(string=w684) -> (number=w686:dbl)  [unwired: 3 in, 1 out]
            n397 = Bundle By Name(cluster=w683, "Injection 1 (Seconds)"=w687, "Injection 2 (Seconds)"=w686) -> (w682:T4)
          }
          frame 53 {
            n398 = Fract/Exp String To Number(string=w690) -> (number=w693:dbl)  [unwired: 3 in, 1 out]
            n399 = Fract/Exp String To Number(string=w691) -> (number=w692:dbl)  [unwired: 3 in, 1 out]
            n400 = Bundle By Name(cluster=w689, "Injection 1 (Seconds)"=w693, "Injection 2 (Seconds)"=w692) -> (w688:T4)
          }
          frame 54 {
            n401 = Fract/Exp String To Number(string=w696) -> (number=w699:dbl)  [unwired: 3 in, 1 out]
            n402 = Fract/Exp String To Number(string=w697) -> (number=w698:dbl)  [unwired: 3 in, 1 out]
            n403 = Bundle By Name(cluster=w695, "Injection 1 (Seconds)"=w699, "Injection 2 (Seconds)"=w698) -> (w694:T4)
          }
          frame 55 {
            n404 = Fract/Exp String To Number(string=w702) -> (number=w705:dbl)  [unwired: 3 in, 1 out]
            n405 = Fract/Exp String To Number(string=w703) -> (number=w704:dbl)  [unwired: 3 in, 1 out]
            n406 = Bundle By Name(cluster=w701, "Injection 1 (Seconds)"=w705, "Injection 2 (Seconds)"=w704) -> (w700:T4)
          }
          frame 56 {
            n407 = Fract/Exp String To Number(string=w709) -> (number=w711:dbl)  [unwired: 3 in, 1 out]
            n408 = Fract/Exp String To Number(string=w708) -> (number=w710:dbl)  [unwired: 3 in, 1 out]
            n409 = Bundle By Name(cluster=w707, "Injection 1 (Seconds)"=w711, "Injection 2 (Seconds)"=w710) -> (w706:T4)
          }
        }
      }
      "Watering Times Output" <- w355
    }
  }
  "Error Out" <- "Error In"
